vi "Create.vi"(8 "error in (no error)":errorcluster) -> (0 "error out":errorcluster, 3 "Excel out":refnum<class "Excel.lvclass">)   [LabVIEW 2016, in "Excel.lvclass"]
doc: "Creates an Excel object which contains .net references for interfacing with Excel.\n\nThis VI does not actually open Excel which should be done later with the \"Open\" VI."
uses:
  Excel.lvclass
  Excel.lvclass/Excel.ctl
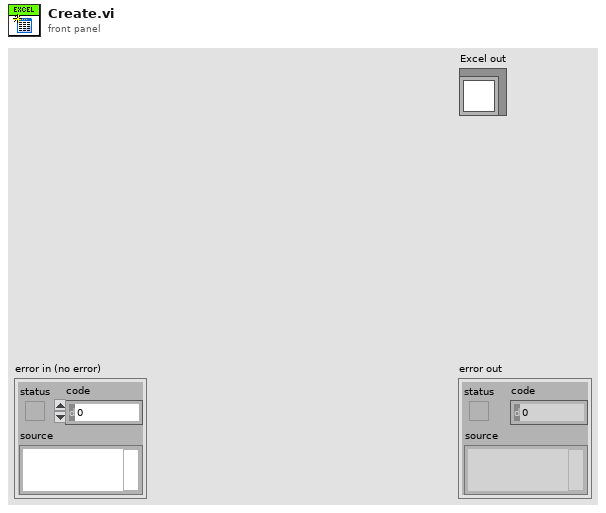
[diagram p1: front panel]
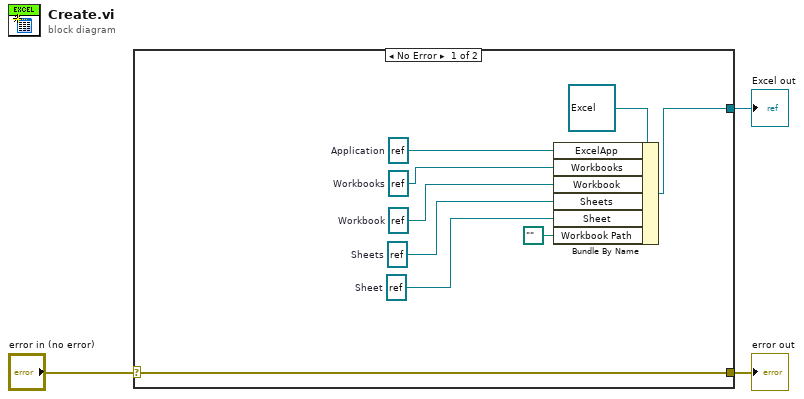
[diagram p0: block diagram]
diagram:
  n1 = case shown="No Error" "error in (no error)" {
    selector: "error in (no error)" -> [w12 w13]
    tunnel: [w12 w13] -> w2
    tunnel: [w10 _] -> w1
    frame No Error {
      w5 = refnum<k7> refnum  # Sheet
      w6 = refnum<k7> refnum  # Sheets
      w7 = refnum<k7> refnum  # Workbook
      w8 = refnum<k7> refnum  # Workbooks
      w9 = refnum<k7> refnum  # Application
      n2 = Bundle By Name(cluster=refnum<class "Excel.lvclass"> refnum ("Excel.lvclass"), "ExcelApp"=w9, "Workbooks"=w8, "Workbook"=w7, "Sheets"=w6, "Sheet"=w5, "Workbook Path"=path "") -> (w10:refnum<class "Excel.lvclass">)
    }
    frame Error {
    }
  }
  "error out" <- w2
  "Excel out" <- w1
